vi "vPage_9234x1_CHx4.vi"() -> ()   [LabVIEW 2022 SP3]
uses:
  <vilib>/Utility/sysdir.llb/System Directory Type.ctl
  <vilib>/express/express analysis/Spectral/Block/exnSpectralBlock spectral measurements peak poly.vi
  <vilib>/express/express analysis/Spectral/Block/exnSpectralBlock spectral measurements peak DDT.vi
  <vilib>/express/express analysis/Spectral/XNode/ExpressSpectralMeasurementsBlockNode.xnode
panel:
  out "C1":i32
  in  "Show_FFT":bool
  in  "Show":bool
  in  "¸ê®Æ§¨\nµù°O>":string
  in  "Filter(Hz)\nLow-Cut":dbl=10.0
  out "DAQ Stoped":bool
  in  "SW \n(C1)":bool[](array[boolean])=[TRUE, TRUE, TRUE, TRUE, TRUE, TRUE, TRUE, TRUE]
  in  "Sample \nto Read":i32=25600
  in  "Sample\nRate":dbl=25600.0
  in  "Enable Saving":bool
  in  "Stop":bool
  out "C1-Save":bool
  out "C1-Trigger":bool
  out "C1-All":dynamicdata(graph)
  out "Statistics":T1(graph)
  out "C1-0":dynamicdata(graph)
  out "C1-2":dynamicdata(graph)
  out "C1-1":dynamicdata(graph)
  out "C1-3":dynamicdata(graph)
  # "使用前請先確認 \nDAQ 擷取卡設定"
  # "本頁畫面顯示為 觸發後訊號"
  # "FFT Filter by useing High-pass with Lower Cut-Off (Hz)"
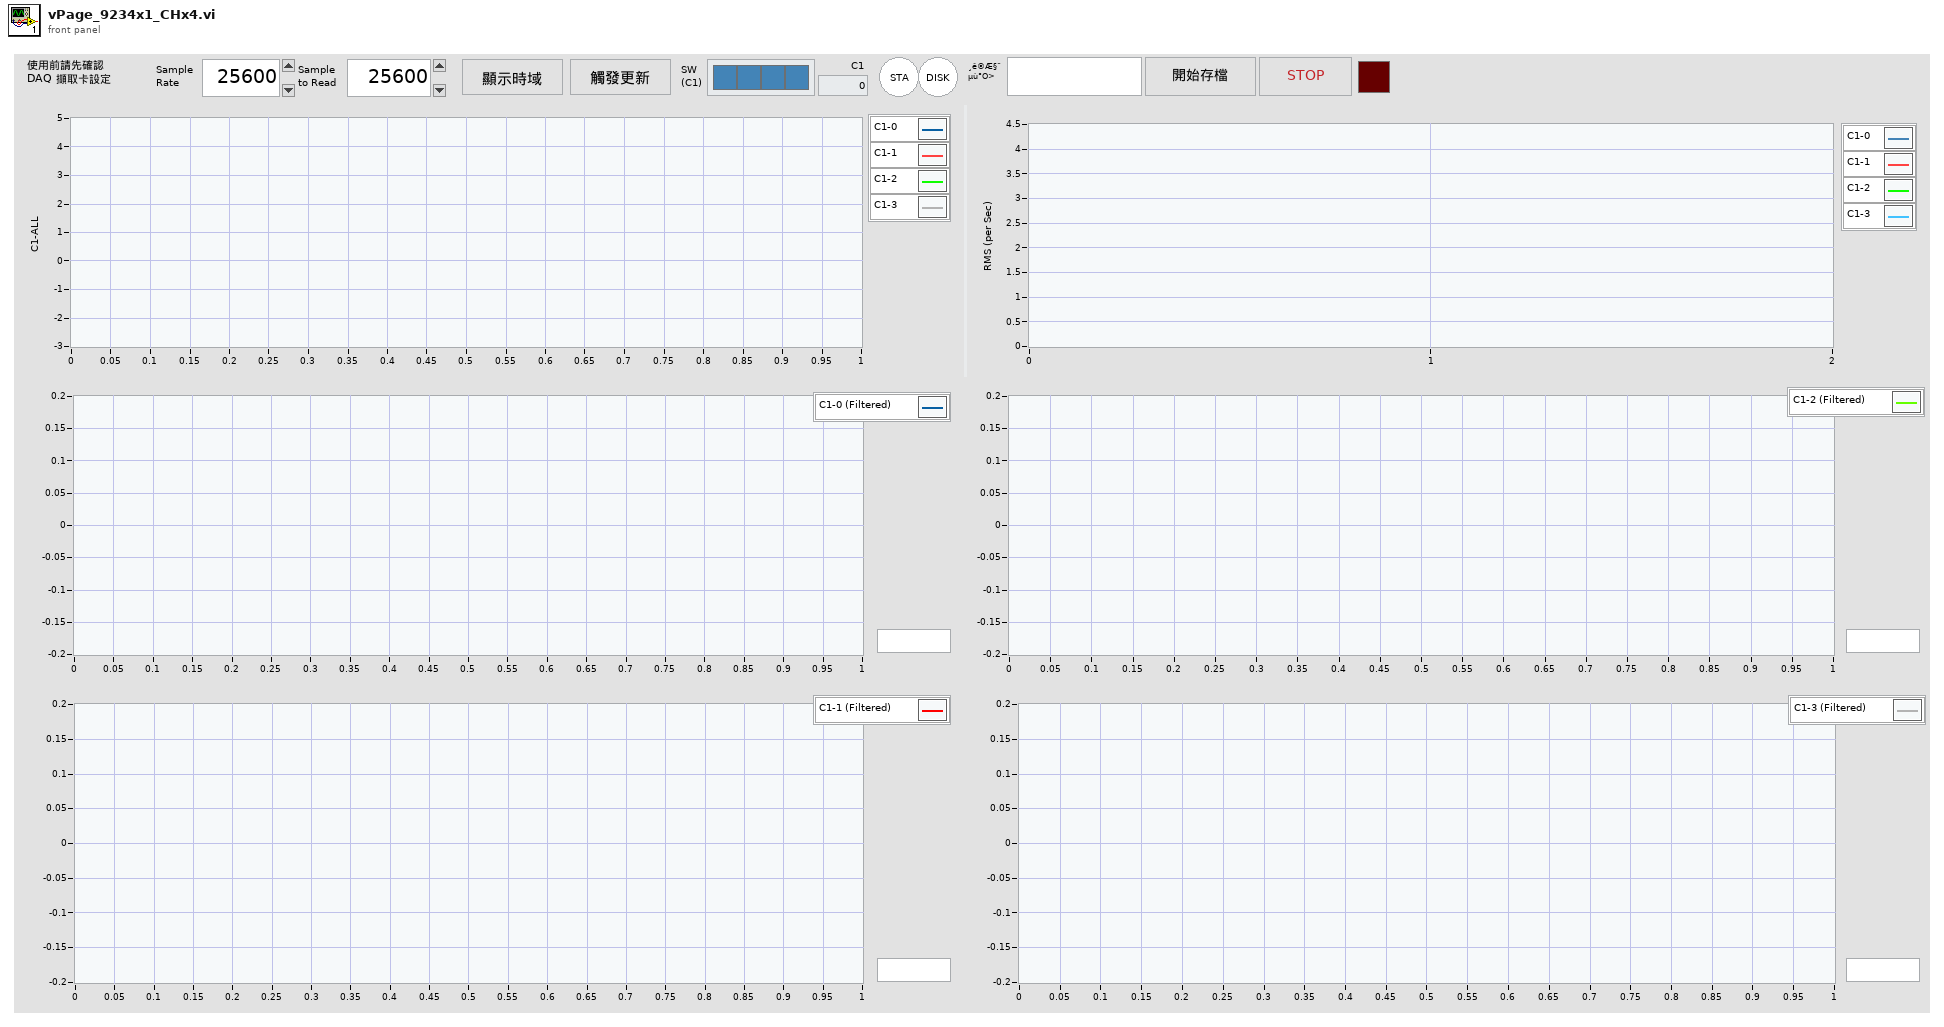
[diagram p1: front panel]
types:
  T1 = cluster{"Array[0]":dbl, "Array[1]":dbl, "Array[2]":dbl, "Array[3]":dbl}
  T2 = cluster{"Array[0]":dbl, "Array[1]":dbl, "Array[2]":dbl, "Array[3]":dbl}[]
  T3 = enum8{"Enabled", "Disabled", "Disabled and Grayed Out"}
  T4 = typedef "System Directory Type.ctl" = i32
  T5 = cluster{"task out":refnum<k21>, "data":dynamicdata}
  T6 = cluster{"averaging mode":u16, "weighting mode":u16, "number of averages":u32}
  T7 = cluster{"dB On (F)":bool, "unwrap phase (F)":bool, "convert to degree (F)":bool}
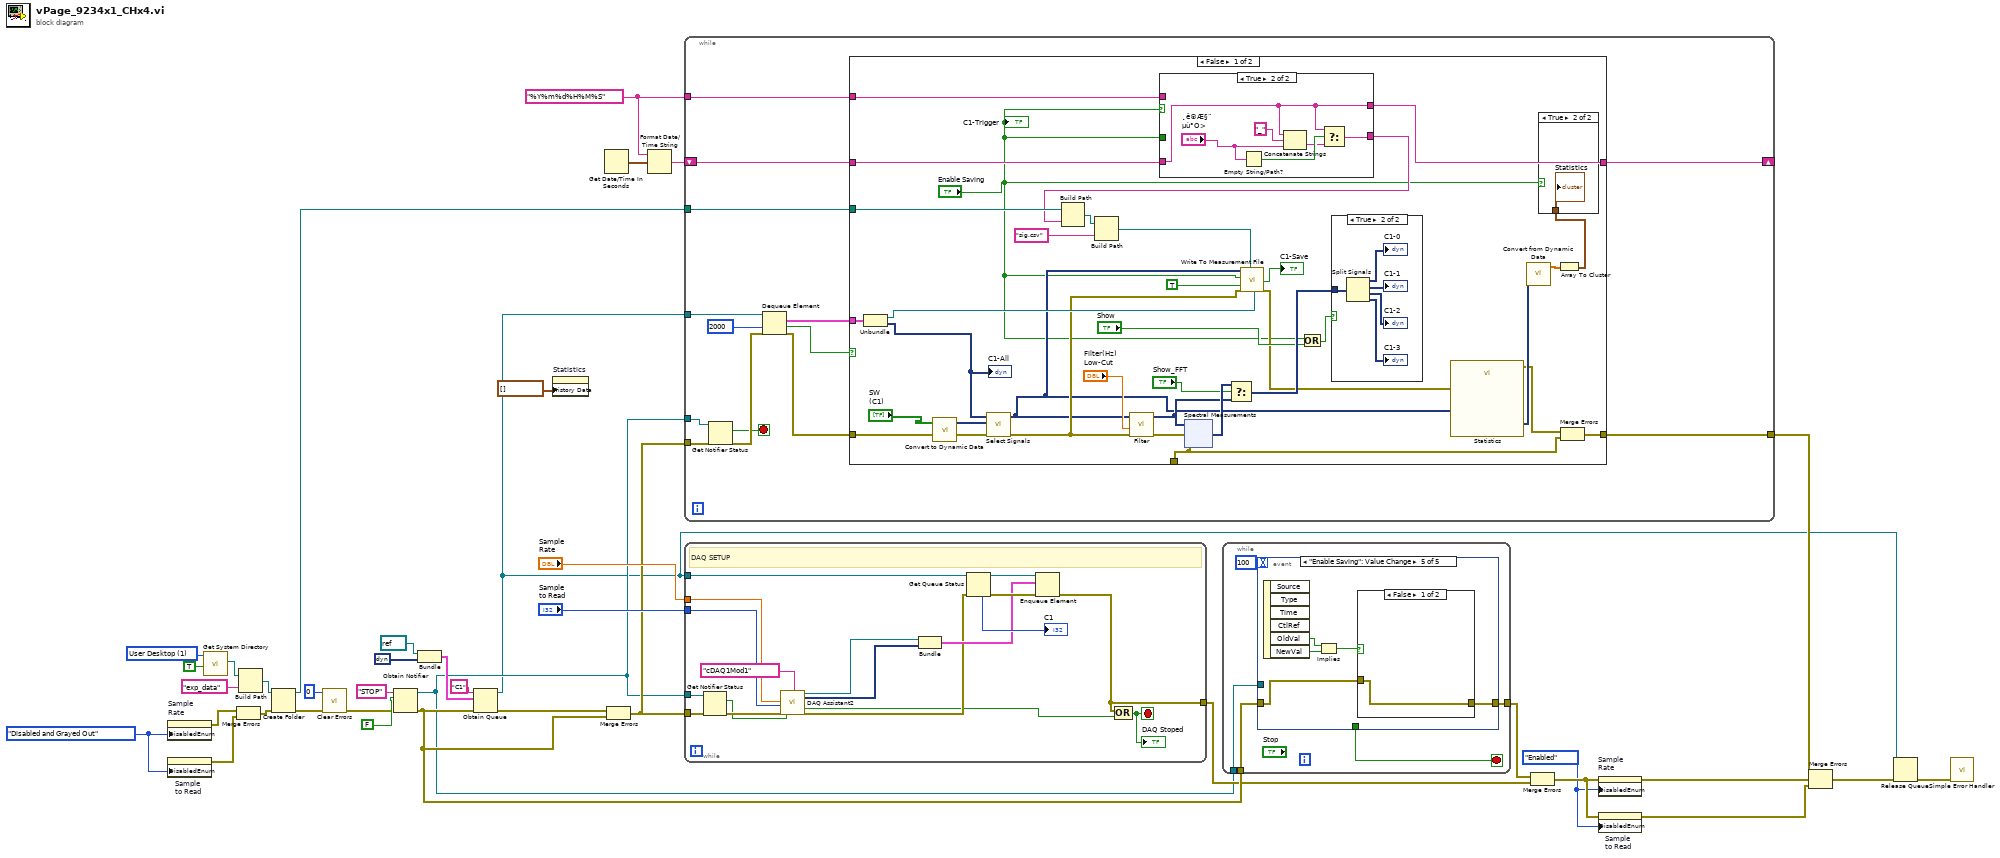
[diagram p0: block diagram]
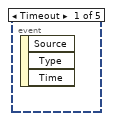
[diagram p2: hidden frame]
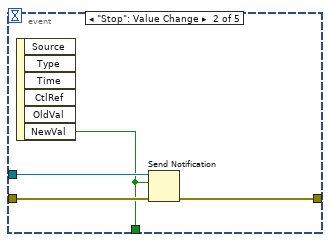
[diagram p3: hidden frame]
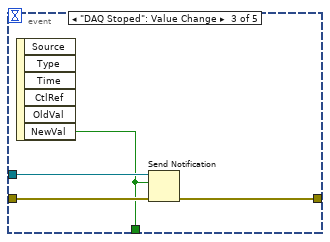
[diagram p4: hidden frame]
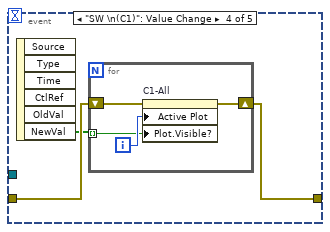
[diagram p5: hidden frame]
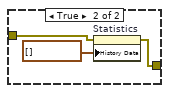
[diagram p6: hidden frame]
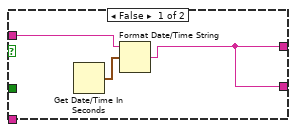
[diagram p9: hidden frame]
diagram:
  w8 = T3."Enabled" ("Disabled")
  w13 = T3."Disabled and Grayed Out" ("Disabled")
  w14 = "%Y%m%d%H%M%S" ("time format string (%c)")
  w24 = T4 1 items=["User Home"=0, "User Desktop"=1, "User Documents"=2, "User Application Data"=3, "User Preferences"=4, "User Temporary"=5, "Public Documents"=6, "Public Application Data"=7, "Public Preferences"=8, "Public Cache"=13, "System Core Libraries"=9, "System Installed Libraries"=10, "Application Files"=11, "Boot Volume Root"=12] ("system directory type")
  n1 = property on="Sample\nRate" class="DigNum (strict)"("DisabledEnum"=w13) -> (error out=w12:errorcluster)  [unwired: 2 in, 1 out]
  n2 = property on="Sample \nto Read" class="DigNum (strict)"("DisabledEnum"=w13) -> (error out=w10:errorcluster)  [unwired: 2 in, 1 out]
  n3 = call <vilib>:"Get System Directory.vi"("create directory if not found? (F)"=TRUE, "system directory type"=w24) -> ("system directory"=w26:path)  [unwired: 9 in]
  n4 = Merge Errors(w12, w10) -> (w11:errorcluster)
  n5 = Build Path(base path=w26, name or relative path="exp_data") -> (appended path=w20:path)
  n6 = Create Folder(path (use dialog)=w20, error in=w11) -> (created path=w19:path, error out=w22:errorcluster)  [unwired: 1 in, 1 out]
  n7 = call <vilib>:"Clear Errors.vi"("error in (no error)"=w22, "specific error code to clear (0: all)"=0) -> ("error out"=w21:errorcluster)  [unwired: 4 in, 1 out]
  n8 = Obtain Notifier(name (unnamed)="STOP", notification data type=FALSE, error in (no error)=w21) -> (notifier out=w15:refnum<notifier>, error out=w18:errorcluster)  [unwired: 1 in, 1 out]
  n9 = Bundle("task out"=refnum<k21> refnum, "data"=dynamicdata []) -> (w31:T5)  [unwired: 1 in]
  n10 = Obtain Queue(name (unnamed)="C1", element data type=w31, error in (no error)=w18) -> (queue out=w2:refnum<queue>, error out=w39:errorcluster)  [unwired: 2 in, 1 out]
  n11 = property on="Statistics" class="WFChart (strict)"("History Data"=T2 []) -> ()  [unwired: 2 in, 2 out]
  n12 = Get Date/Time In Seconds() -> (seconds since 1Jan1904=w29:timestamp)
  n13 = Merge Errors(w39, w18) -> (w30:errorcluster)
  n14 = Format Date/Time String(time format string (%c)=w14, seconds (now)=w29) -> (date/time string=w28:string)  [unwired: 1 in]
  n15 = while {
    tunnel: w30 -> [w53]
    tunnel: w15 -> [w51]
    tunnel: w2 -> [w50]
    shift-right: [w40] -> _
    shift-left: w28 -> [w44]
    tunnel: w19 -> [w45]
    tunnel: [w41] -> w3
    tunnel: w14 -> [w43]
    stop <- w48 stop-if-true
    n16 = Get Notifier Status(notifier=w51, error in (no error)=w53) -> (current notification=w48:bool, error out=w52:errorcluster)  [unwired: 3 out]
    n17 = Dequeue Element(queue=w50, timeout in ms (-1)=2000, error in (no error)=w52) -> (element=w46:T5, timed out?=w47:bool, error out=w42:errorcluster)  [unwired: 1 out]
    n18 = case shown="False" w47 {
      tunnel: w46 -> [w85 _]
      tunnel: w42 -> [w84 w113]
      tunnel: [w75 _] -> _
      tunnel: w44 -> [w81 w114]
      tunnel: [w80 w114] -> w40
      tunnel: w45 -> [w79 _]
      tunnel: [w74 w113] -> w41
      tunnel: w43 -> [w67 _]
      frame False {
        n19 = Unbundle(w85) -> ("task out"=w83:refnum<k21>, "data"=w63:dynamicdata)
        "C1-All" <- w63
        n20 = call "Convert to Dynamic Data"("Array"="SW \n(C1)") -> ("Dynamic Data Type"=w71:dynamicdata)  [unwired: 3 in]
        n21 = call "Select Signals"("error in (no error)"=w84, "Selector Input"=w71, "Signals"=w63) -> ("error out"=w82:errorcluster, "Signal Out"=w60:dynamicdata)  [unwired: 7 in]
        n22 = call "Filter"("error in (no error)"=w82, "Lower Cut-Off"="Filter(Hz)\nLow-Cut", "Signal"=w60) -> ("error out"=w87:errorcluster, "Filtered Signal"=w72:dynamicdata)  [unwired: 7 in]
        n23 = case shown="True" "Enable Saving" {
          tunnel: [w94 w98] -> w80
          tunnel: "Enable Saving" -> [_ _]
          tunnel: w81 -> [_ w98]
          tunnel: [w94 w100] -> w68
          tunnel: w67 -> [w95 _]
          frame False {
            n24 = Get Date/Time In Seconds() -> (seconds since 1Jan1904=w96:timestamp)
            n25 = Format Date/Time String(time format string (%c)=w95, seconds (now)=w96) -> (date/time string=w94:string)  [unwired: 1 in]
          }
          frame True {
            n26 = Empty String/Path?(string/path="¸ê®Æ§¨\nµù°O>") -> (empty?=w102:bool)
            n27 = Concatenate Strings(w98, "_" ("string"), "¸ê®Æ§¨\nµù°O>") -> (w101:string)
            n28 = Select(t=w98, s=w102, f=w101) -> (s? t:f=w100:string)
          }
        }
        n29 = Build Path(base path=w79, name or relative path=w68) -> (appended path=w78:path)
        n30 = Build Path(base path=w78, name or relative path="sig.csv") -> (appended path=w76:path)
        n31 = xnode ("Spectral Measurements")("Signals"=w72, "error in (no error)"=w87) -> ("FFT - (Peak)"=w73:dynamicdata, "error out"=w75:errorcluster)  [unwired: 1 out]
        n32 = Select(t=w73, s="Show_FFT", f=w72) -> (s? t:f=w70:dynamicdata)
        n33 = call "Write To Measurement File"("Signals"=w60, "Enable"="Enable Saving", "new_file"=TRUE, "error in (no error)"=w82, "Filename"=w76, "DAQmx Task"=w83) -> ("Saving Data"=→"C1-Save":bool, "error out"=w56:errorcluster)  [unwired: 11 in, 1 out]
        n34 = Or(x="Enable Saving", y="Show") -> (x .or. y?=w66:bool)
        n35 = case shown="True" w66 {
          tunnel: w70 -> [_ w90]
          frame False {
          }
          frame True {
            n36 = Split Signals(w90) -> (→"C1-0":dynamicdata, →"C1-1":dynamicdata, →"C1-2":dynamicdata, →"C1-3":dynamicdata)  [unwired: 4 in]
          }
        }
        n37 = call "Statistics"("Signals"=w60, "error in (no error)"=w56) -> ("RMS"=w59:dynamicdata, "error out"=w55:errorcluster)  [unwired: 24 in]
        n38 = call "Convert from Dynamic Data"("Dynamic Data Type"=w59) -> ("Array"=w58:dbl[])  [unwired: 3 in]
        n39 = Array To Cluster(array=w58) -> (cluster=w57:T1)
        n40 = case shown="True" "Enable Saving" {
          tunnel: w57 -> [_ w88]
          frame False {
          }
          frame True {
            "Statistics" <- w88
          }
        }
        n41 = Merge Errors(w55, w75) -> (w74:errorcluster)
        "C1-Trigger" <- "Enable Saving"
      }
      frame True {
      }
    }
  }
  n42 = while {
    tunnel: [w131] -> w16
    tunnel: w2 -> [w128]
    tunnel: w30 -> [w127]
    tunnel: w15 -> [w126]
    tunnel: "Sample \nto Read" -> [w120]
    tunnel: "Sample\nRate" -> [w121]
    stop <- w129 stop-if-true
    # "DAQ SETUP"
    n43 = Get Notifier Status(notifier=w126, error in (no error)=w127) -> (current notification=w119:bool, error out=w123:errorcluster)  [unwired: 3 out]
    n44 = call "DAQ Assistant2"("rate"=w121, "number of samples"=w120, "error in"=w123, "stop (F)"=w119, "device name"=tag "cDAQ1Mod1") -> ("task out"=w117:refnum<k21>, "data"=w116:dynamicdata, "stopped"=w118:bool, "error out"=w122:errorcluster)  [unwired: 11 in]
    n45 = Bundle("task out"=w117, "data"=w116) -> (w124:T5)  [unwired: 1 in]
    n46 = Get Queue Status(queue=w128, error in (no error)=w122) -> (queue out=w125:refnum<queue>, error out=w132:errorcluster, # elements in queue=→"C1":i32)  [unwired: 1 in, 5 out]
    n47 = Enqueue Element(queue=w125, element=w124, error in (no error)=w132) -> (error out=w131:errorcluster)  [unwired: 1 in, 2 out]
    n48 = Compound Arithmetic op=OR(w131, w118) -> (w129:bool)
    "DAQ Stoped" <- w129
  }
  n49 = while {
    tunnel: w18 -> [w137]
    tunnel: [w136] -> w17
    tunnel: w15 -> [w135]
    stop <- w134 stop-if-true
    n50 = event shown="[4] \"Enable Saving\": Value Change" {
      selector: _ -> [_ _ _ _ _]
      dyn-events: _ -> [_ _ _ _ _]
      timeout: 100 -> [_ _ _ _ _]
      tunnel: w137 -> [_ w141 w145 w148 w155]
      tunnel: [_ w140 w144 w147 w154] -> w136
      tunnel: w135 -> [_ w139 w143 _ _]
      tunnel: [_ w138 w142 _ _] -> w134
      event Timeout {
        n51 = event-data() -> ()  [unwired: 1 in, 3 out]
      }
      event "Stop": Value Change {
        n52 = event-data() -> ("NewVal"=w138:bool)  [unwired: 1 in, 5 out]
        n53 = Send Notification(notification=w138, notifier=w139, error in (no error)=w141) -> (error out=w140:errorcluster)  [unwired: 1 out]
      }
      event "DAQ Stoped": Value Change {
        n54 = event-data() -> ("NewVal"=w142:bool)  [unwired: 1 in, 5 out]
        n55 = Send Notification(notification=w142, notifier=w143, error in (no error)=w145) -> (error out=w144:errorcluster)  [unwired: 1 out]
      }
      event "SW \n(C1)": Value Change {
        n56 = event-data() -> ("NewVal"=w146:bool[])  [unwired: 1 in, 5 out]
        n57 = for {
          shift-right: [w149] -> w147
          shift-left: w148 -> [w151]
          tunnel: w146 -> [w150] mode=indexing
          i -> [w152]
          n58 = property on="C1-All" class="WFGraph (strict)"(error in=w151, "Active Plot"=w152, "Plot.Visible?"=w150) -> (error out=w149:errorcluster)  [unwired: 1 in, 1 out]
        }
      }
      event "Enable Saving": Value Change {
        n59 = event-data() -> ("OldVal"=w156:bool, "NewVal"=w157:bool)  [unwired: 1 in, 4 out]
        n60 = Implies(1:w157, 2:w156) -> (0:w153:bool)
        n61 = case shown="False" w153 {
          tunnel: w155 -> [w158 w160]
          tunnel: [w158 w159] -> w154
          frame False {
          }
          frame True {
            n62 = property on="Statistics" class="WFChart (strict)"(error in=w160, "History Data"=T2 []) -> (error out=w159:errorcluster)  [unwired: 1 in, 1 out]
          }
        }
      }
    }
  }
  n63 = Merge Errors(w17, w16) -> (w9:errorcluster)
  n64 = property on="Sample\nRate" class="DigNum (strict)"(error in=w9, "DisabledEnum"=w8) -> (error out=w7:errorcluster)  [unwired: 1 in, 1 out]
  n65 = property on="Sample \nto Read" class="DigNum (strict)"(error in=w9, "DisabledEnum"=w8) -> (error out=w6:errorcluster)  [unwired: 1 in, 1 out]
  n66 = Merge Errors(w3, w7, w6) -> (w4:errorcluster)
  n67 = Release Queue(queue=w2, error in (no error)=w4) -> (error out=w5:errorcluster)  [unwired: 1 in, 2 out]
  n68 = call <vilib>:"Simple Error Handler.vi"("error in (no error)"=w5) -> ()  [unwired: 4 in, 5 out]
